vi "1_7.vi"() -> ()   [LabVIEW 2020]
panel:
  out "Boolean":bool
  in  "C":bool
  in  "B":bool
  in  "A":bool
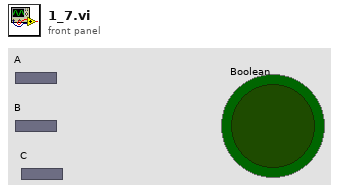
[diagram p1: front panel]
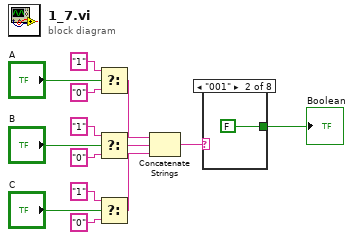
[diagram p0: block diagram]
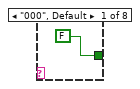
[diagram p2: hidden frame]
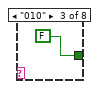
[diagram p3: hidden frame]
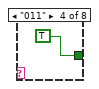
[diagram p4: hidden frame]
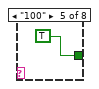
[diagram p5: hidden frame]
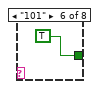
[diagram p6: hidden frame]
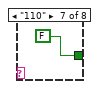
[diagram p7: hidden frame]
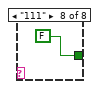
[diagram p8: hidden frame]
diagram:
  n1 = Select(t="1", s="A", f="0") -> (s? t:f=w5:string)
  n2 = Select(t="1", s="B", f="0") -> (s? t:f=w4:string)
  n3 = Select(t="1", s="C", f="0") -> (s? t:f=w3:string)
  n4 = Concatenate Strings(w5, w4, w3) -> (w2:string)
  n5 = case shown="\"001\"" w2 {
    tunnel: [FALSE ("Boolean") FALSE ("Boolean") FALSE ("Boolean") TRUE TRUE TRUE FALSE ("Boolean") FALSE ("Boolean")] -> w1
    frame "000", Default {
    }
    frame "001" {
    }
    frame "010" {
    }
    frame "011" {
    }
    frame "100" {
    }
    frame "101" {
    }
    frame "110" {
    }
    frame "111" {
    }
  }
  "Boolean" <- w1
